vi "Écrire_Instruction.vi"(8 "error in (no error)":errorcluster caption="entrée d'erreur (pas d'erreur)", 10 "Instruction":string="import sys\nimport numpy as np\nfrom sklearn.model_selection import {splitter_name}\n\ndef exec(n_splits,X,y=None,groups=None):\n    X,y = np.array(X),np.array(y)\n    groups = np.array(groups)\n    try:\n        import json\n        splitter = {splitter_name}({params})\n        l_train_index = []\n        l_test_index = []\n        for train_index,test_index in splitter.split(X,y,groups):\n            l_train_index.append(train_index.tolist())\n            l_test_index.append(test_index.tolist())\n        return json.dumps({'train_index':l_train_index,\n                'test_index':l_test_index}).replace(' ','')\n    except:\n        erreur = sys.exc_info()\n        typerr = u\"%s\" % (erreur[0])\n        typerr = typerr[typerr.find(\"'\")+1:typerr.rfind(\"'\")]\n        msgerr = u\"%s\" % (erreur[1])\n        message = str('/!\\\\ {0} : {1}'. format(typerr,msgerr))\n        return message", 11 "Splitter en entrée":refnum<class "Splitter.lvclass">) -> (0 "error out":errorcluster caption="sortie d'erreur", 3 "Splitter en sortie":refnum<class "Splitter.lvclass">)   [LabVIEW 2020, in "Splitter.lvclass"]
uses:
  Splitter.lvclass
  Splitter.lvclass/Splitter.ctl
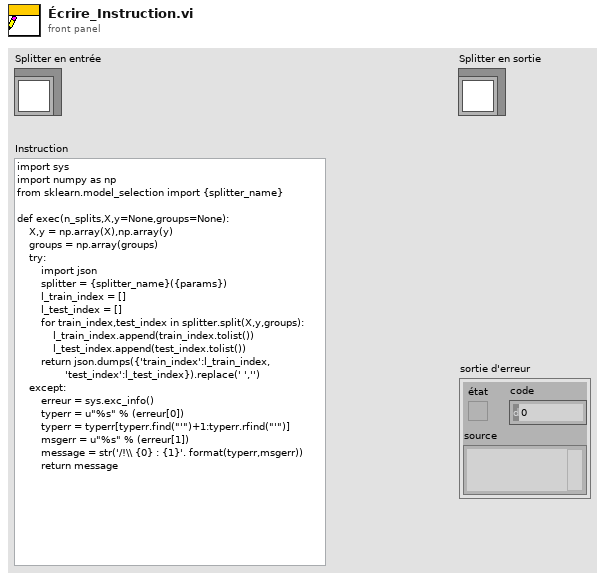
[diagram p1: front panel]
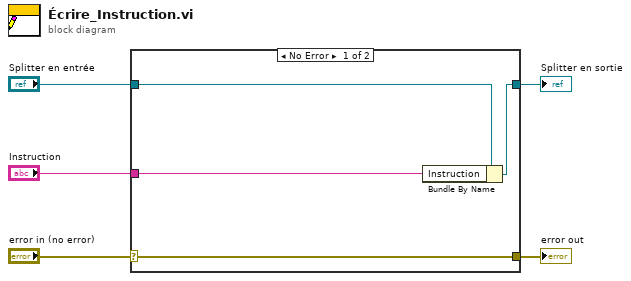
[diagram p0: block diagram]
diagram:
  n1 = case shown="No Error" "error in (no error)" {
    selector: "error in (no error)" -> [w9 w10]
    tunnel: [w9 w10] -> w4
    tunnel: [w7 w11] -> w2
    tunnel: "Splitter en entrée" -> [w8 w11]
    tunnel: "Instruction" -> [w6 _]
    frame No Error {
      n2 = Bundle By Name(cluster=w8, "Instruction"=w6) -> (w7:refnum<class "Splitter.lvclass">)
    }
    frame Error {
    }
  }
  "error out" <- w4
  "Splitter en sortie" <- w2
